vi "Text File to String Array.vi"(1 "file (use dialog)":path=path "C:/Users/Nick/Documents/Test.txt") -> (0 "Array":string[](array[string]))   [LabVIEW 2014]
panel:
  out "text":string
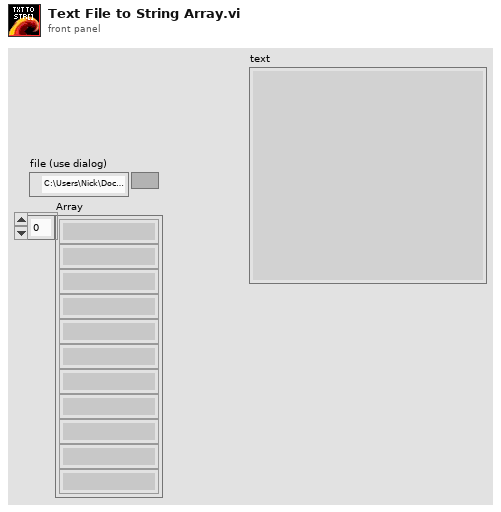
[diagram p1: front panel]
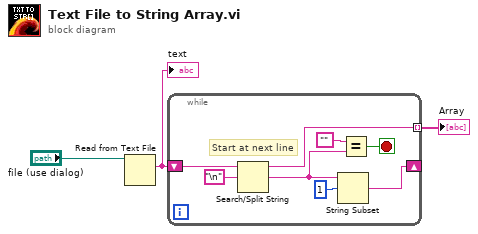
[diagram p0: block diagram]
diagram:
  n1 = Read from Text File(file (use dialog)="file (use dialog)") -> (text=w3:string)  [unwired: 3 in, 3 out]
  "text" <- w3
  n2 = while {
    shift-right: [w6] -> _
    shift-left: w3 -> [w9]
    tunnel: [w5] -> w1 mode=indexing
    stop <- w7 stop-if-true
    # "Start at next line"
    n3 = Search/Split String(string=w9, search string/char (-)="\n") -> (substring before match=w5:string, match + rest of string=w4:string)  [unwired: 1 in, 1 out]
    n4 = String Subset(string=w4, offset (0)=1) -> (substring=w6:string)  [unwired: 1 in]
    n5 = Equal?(x="", y=w4) -> (x = y?=w7:bool)
  }
  "Array" <- w1
